vi "Record_End.vi"(8 "error in":errorcluster, 9 "Settings in":T4={"Harware Configuration"={"Camera"="cam1", "Frames Per Second"=15, "Simulate Recording"=FALSE, "Simulated Recording Sample"=path "", "Timestamp Method"=enum."Camera Timestamp"}, "Base Recording Path"=path "", "Type Of Recording"="", "Recording Codec"="", "TrackingSettings"={"Max Radius"=0, "Threshold"=160.0, "ROI"={"Left"=0, "Top"=0, "Right"=0, "Bottom"=0, "Rotation"=0.0}}, "Calibration"={"Pixel Width (X)"=1.0, "Pixel Height (Y)"=1.0}, "Broadcast Length"=0} {"Broadcast Length" min=0; "TrackingSettings"."ROI"."Rotation" format="%.2f"; "TrackingSettings"."ROI"."Left" scale=0.0..1024.0; "TrackingSettings"."ROI"."Right" scale=0.0..1024.0; "TrackingSettings"."Threshold" scale=0.0..255.0}, 10 "Data Queue":refnum<queue>, 11 "Recording Data":T1) -> (0 "error out":errorcluster, 2 "Data Queue Out":refnum<queue>, 3 "Recording Data 2":T1)   [LabVIEW 2017, in "ImageAcquisitionLibrary.lvlib"]
uses:
  ImageAcquisitionLibrary.lvlib
  Settings/Settings.ctl
  <vilib>/userdefined/High Color/IMAQdx.ctl
  Tracking/TrackingSettings.ctl
  Settings/Calibration.ctl
  Acquisition/AcquireData.ctl
  RecordingData.ctl
  <vilib>/vision/Image Controls.llb/IMAQ Image.ctl
  <vilib>/vision/Avi.llb/IMAQ AVI2 Refnum.ctl
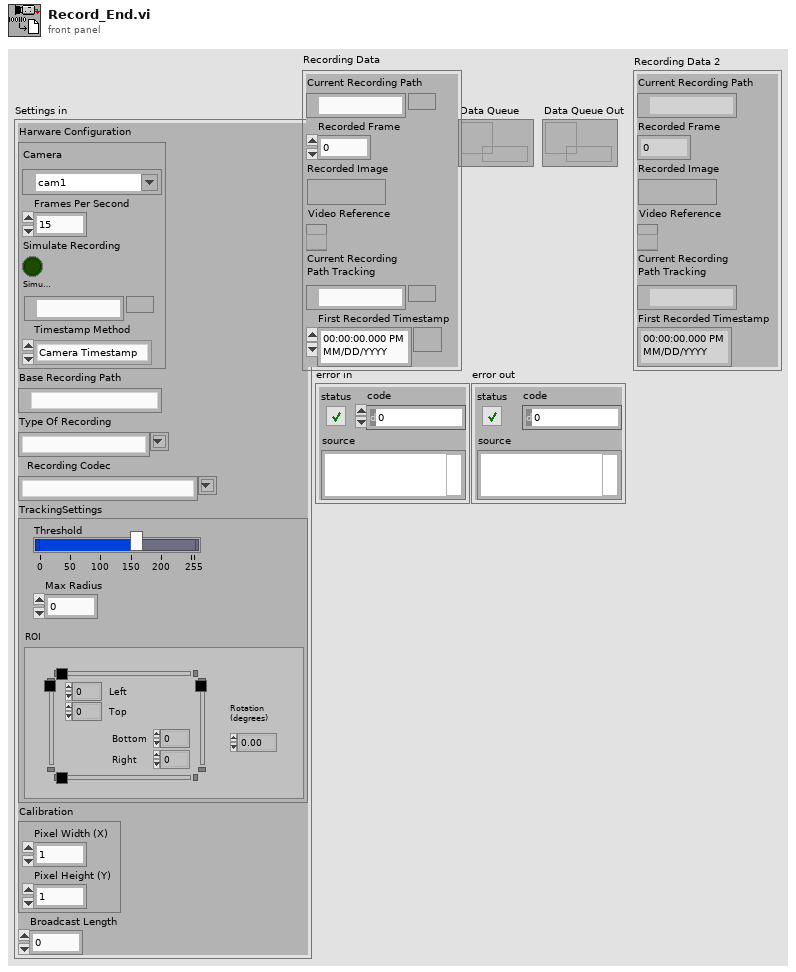
[diagram p1: front panel]
types:
  T1 = typedef "ImageAcquisitionLibrary.lvlib/RecordingData.ctl" = cluster{"Current Recording Path":path, "Recorded Frame":i32, "Recorded Image":T2, "Video Reference":T3, "Current Recording \nPath Tracking":path, "First Recorded Timestamp":timestamp}
  T2 = typedef "IMAQ Image.ctl" = refnum<image>
  T3 = typedef "IMAQ AVI2 Refnum.ctl" = refnum<k20>
  T4 = typedef "ImageAcquisitionLibrary.lvlib/Settings.ctl" = cluster{"Harware Configuration":cluster{"Camera":T5, "Frames Per Second":u32, "Simulate Recording":bool, "Simulated Recording Sample":path, "Timestamp Method":enum16{"System Timestamp", "Camera Timestamp", "IMAQdx Timestamp"}}, "Base Recording Path":path, "Type Of Recording":string, "Recording Codec":string, "TrackingSettings":T6, "Calibration":T8, "Broadcast Length":i32}
  T5 = typedef "IMAQdx.ctl" = refnum<k21>
  T6 = typedef "ImageAcquisitionLibrary.lvlib/TrackingSettings.ctl" = cluster{"Max Radius":i32, "Threshold":sgl, "ROI":T7}
  T7 = typedef "IMAQ Rectangle" = cluster{"Left":i32, "Top":i32, "Right":i32, "Bottom":i32, "Rotation":dbl}
  T8 = typedef "ImageAcquisitionLibrary.lvlib/Calibration.ctl" = cluster{"Pixel Width (X)":dbl, "Pixel Height (Y)":dbl}
  T9 = typedef "ImageAcquisitionLibrary.lvlib/AcquireData.ctl" = cluster{"Frame Data":cluster{"Image":u32[][], "Timestamp":timestamp, "Image Type":T10, "Dropped Frames":u32}, "Tracking Data":cluster{"Positions":dbl[][], "Timestamp":timestamp}, "Tracked?":bool}
  T10 = typedef "Image Type" = u32
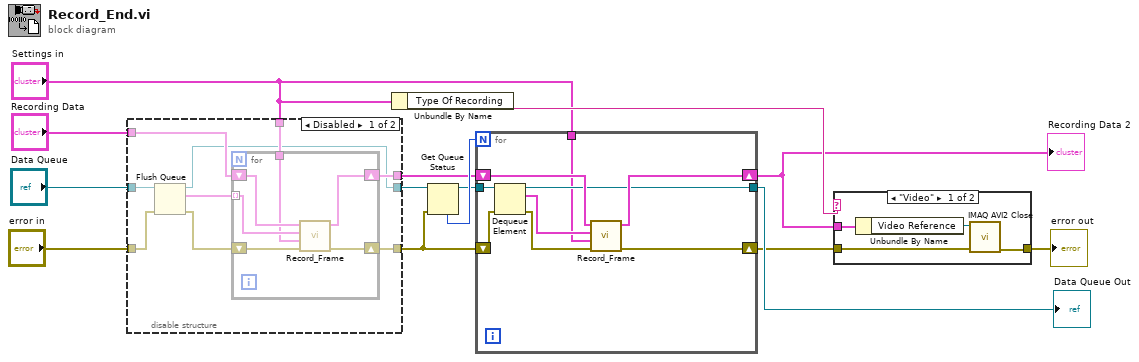
[diagram p0: block diagram]
diagram:
  n1 = disable-structure shown="Disabled" {
    disable-tunnel: "Data Queue" -> [w23 w31]
    disable-tunnel: [w21 w32] -> w2
    disable-tunnel: "Recording Data" -> [w20 w30]
    disable-tunnel: [w19 w30] -> w6
    disable-tunnel: "Settings in" -> [w18 _]
    disable-tunnel: [w17 w31] -> w9
    disable-tunnel: "error in" -> [w16 w32]
    frame Disabled {
      n2 = Flush Queue(queue=w23, error in (no error)=w16) -> (queue out=w17:refnum<queue>, remaining elements=w22:T9[], error out=w15:errorcluster)
      n3 = for {
        tunnel: w22 -> [w26] mode=indexing
        shift-right: [w28] -> w21
        shift-left: w15 -> [w29]
        shift-right: [w25] -> w19
        shift-left: w20 -> [w27]
        tunnel: w18 -> [w24]
        n4 = call "Record_Frame.vi"("error in"=w29, "Settings"=w24, "Image Data"=w26, "Recording Data In"=w27) -> ("error out"=w28:errorcluster, "Recording Data Out"=w25:T1)  [unwired: 6 in]
      }
    }
    frame Enabled {
    }
  }
  n5 = Unbundle By Name("Settings in") -> ("Type Of Recording"=w12:string)
  n6 = Get Queue Status(queue=w9, error in (no error)=w2) -> (queue out=w4:refnum<queue>, # elements in queue=w8:i32)  [unwired: 1 in, 6 out]
  n7 = for {
    N: w8 -> [_]
    shift-right: [w39] -> w7
    shift-left: w6 -> [w40]
    tunnel: w4 -> [w36]
    tunnel: [w35] -> w5
    shift-right: [w41] -> w3
    shift-left: w2 -> [w38]
    tunnel: "Settings in" -> [w33]
    n8 = Dequeue Element(queue=w36, error in (no error)=w38) -> (queue out=w35:refnum<queue>, element=w34:T9, error out=w37:errorcluster)  [unwired: 1 in, 1 out]
    n9 = call "Record_Frame.vi"("error in"=w37, "Settings"=w33, "Image Data"=w34, "Recording Data In"=w40) -> ("error out"=w41:errorcluster, "Recording Data Out"=w39:T1)  [unwired: 6 in]
  }
  "Recording Data 2" <- w7
  "Data Queue Out" <- w5
  n10 = case shown="\"Video\"" w12 {
    tunnel: w3 -> [w42 w46]
    tunnel: [w45 w46] -> w13
    tunnel: w7 -> [w44 _]
    frame "Video" {
      n11 = Unbundle By Name(w44) -> ("Video Reference"=w43:T3)
      n12 = call "IMAQ AVI2 Close"("error in (no error)"=w42, "AVI Refnum"=w43) -> ("error out"=w45:errorcluster)  [unwired: 9 in]
    }
    frame "Snapshot", Default {
    }
  }
  "error out" <- w13
